vi "Read Device ID Type.vi"(8 "error in (no error)":errorcluster, 11 "device data model in":refnum<class "Device Data Model.lvclass">) -> (0 "error out":errorcluster, 2 "read device ID code":u8(ring)=1 items=["None"=0, "Basic Stream"=1, "Regular Stream"=2, "Extended Stream"=3, "Basic Stream/Individual"=129, "Regular Stream/Individual"=130, "Extended Stream/Individual"=131], 3 "device data model out":refnum<class "Device Data Model.lvclass">)   [LabVIEW 2017, in "SubVIs.lvlib" / "Device Data Model.lvclass"]
doc: "Reads the device ID stored in the device data model."
uses:
  <vilib>/Modbus/subvis/Data and Functions/Device Data Model/Device Data Model.lvclass
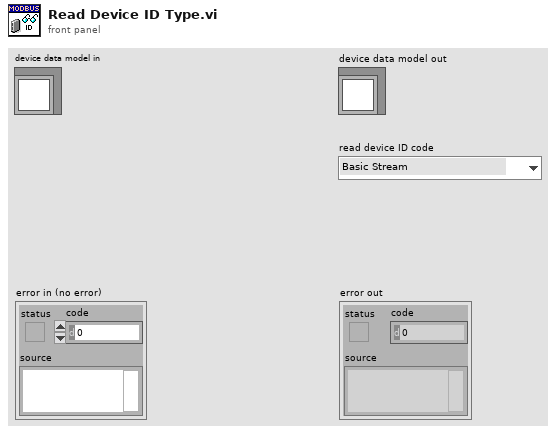
[diagram p1: front panel]
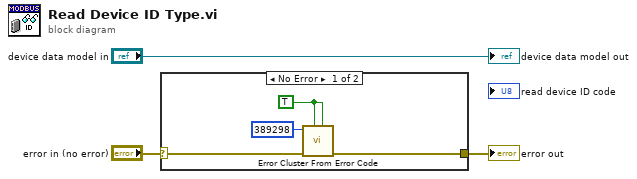
[diagram p0: block diagram]
diagram:
  n1 = case shown="No Error" "error in (no error)" {
    selector: "error in (no error)" -> [w6 w8]
    tunnel: [w7 w8] -> w1
    frame No Error {
      w4 = TRUE ("show call chain? (False)")
      n2 = call <vilib>:"Error Cluster From Error Code.vi"("is warning? (False)"=w4, "show call chain? (False)"=w4, "error in (no error)"=w6, "error code (0)"=389298) -> ("error out"=w7:errorcluster)  [unwired: 5 in]
    }
    frame Error {
    }
  }
  "error out" <- w1
  "device data model out" <- "device data model in"
